vi "eleva.vi"(10 "Position:Top":i32, 11 "Boolean in":refnum<vi>) -> ()   [LabVIEW 2020]
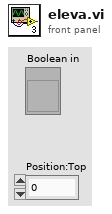
[diagram p1: front panel]
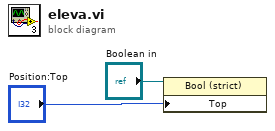
[diagram p0: block diagram]
diagram:
  n1 = property on="Property Node" class="Bool (strict)"(reference="Boolean in", "Top"="Position:Top") -> ()  [unwired: 1 in, 2 out]
